vi "PXI4072 Update UI Status.vi"(8 "error in (no error)":errorcluster, 10 "Instr Status":string, 11 "PXI4072 All UI Refs":T1) -> (0 "error out":errorcluster)   [LabVIEW 2026]
uses:
  App Types/References/PXI4072 All UI References.ctl
  App Types/References/PXI4072 Boolean UI References.ctl
  App Types/References/PXI4072 String UI References.ctl
  App Types/References/PXI4072 Numeric UI References.ctl
  App Types/References/PXI4072 Other UI Rerences.ctl
  Drivers/PXI4072/Types/PXI4072 Settings.ctl
  <instrlib>/niDMM/nidmm.llb/niDMM Function.ctl
  <instrlib>/niDMM/nidmm.llb/niDMM Resolution in Digits.ctl
  App Types/Globals/PXI4072 UI Global Refs.vi
  Drivers/PXI4072/PXI4072.lvlib
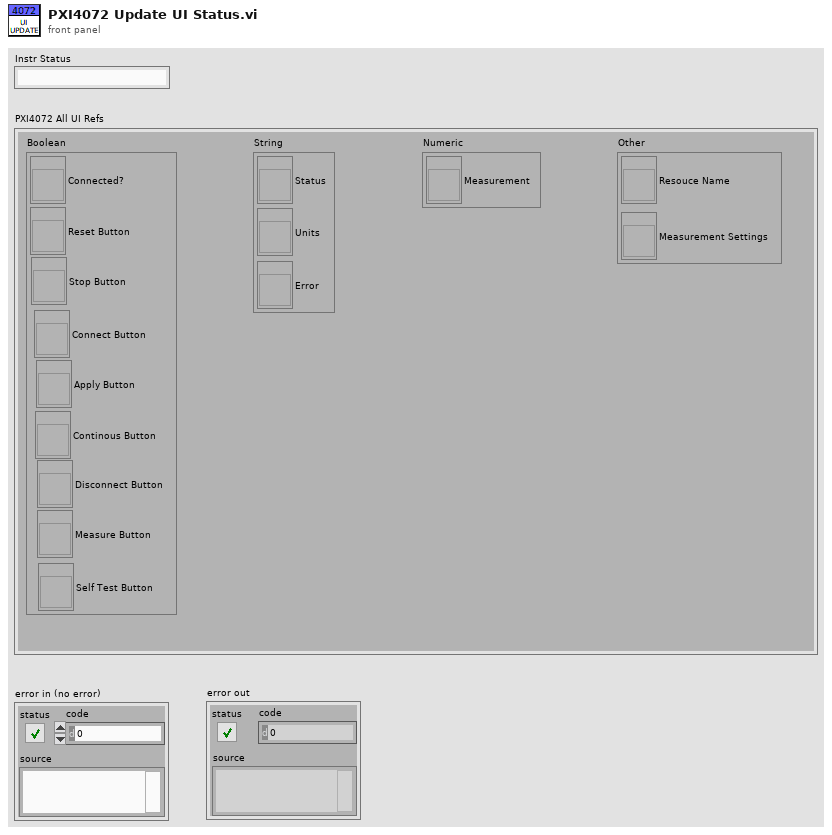
[diagram p1: front panel]
types:
  T1 = typedef "PXI4072 All UI References.ctl" = cluster{"Boolean":T2, "String":T3, "Numeric":T4, "Other":T5}
  T2 = typedef "PXI4072 Boolean UI References.ctl" = cluster{"Connected?":refnum<vi>, "Reset Button":refnum<vi>, "Connect Button":refnum<vi>, "Apply Button":refnum<vi>, "Disconnect Button":refnum<vi>, "Measure Button":refnum<vi>, "Self Test Button":refnum<vi>, "Continous Button":refnum<vi>, "Stop Button":refnum<vi>}
  T3 = typedef "PXI4072 String UI References.ctl" = cluster{"Status":refnum<vi>, "Units":refnum<vi>, "Error":refnum<vi>}
  T4 = typedef "PXI4072 Numeric UI References.ctl" = cluster{"Measurement":refnum<vi>}
  T5 = typedef "PXI4072 Other UI Rerences.ctl" = cluster{"Resouce Name":refnum<vi>, "Measurement Settings":refnum<vi>}
  T6 = enum8{"Enabled", "Disabled", "Disabled and Grayed Out"}
  T7 = typedef "PXI4072.lvlib/PXI4072 Settings.ctl" = cluster{"Function":T8, "Resolution in Digits":T9, "Range":dbl}
  T8 = typedef "niDMM Function.ctl" = enum16{"DC Volts", "AC Volts", "DC Current", "AC Current", "2-wire Resistance", "4-wire Resistance", "Diode", "Frequency", "Period", "AC Volts DC Coupled", "Capacitance", "Inductance", "Temperature"}
  T9 = typedef "niDMM Resolution in Digits.ctl" = dbl
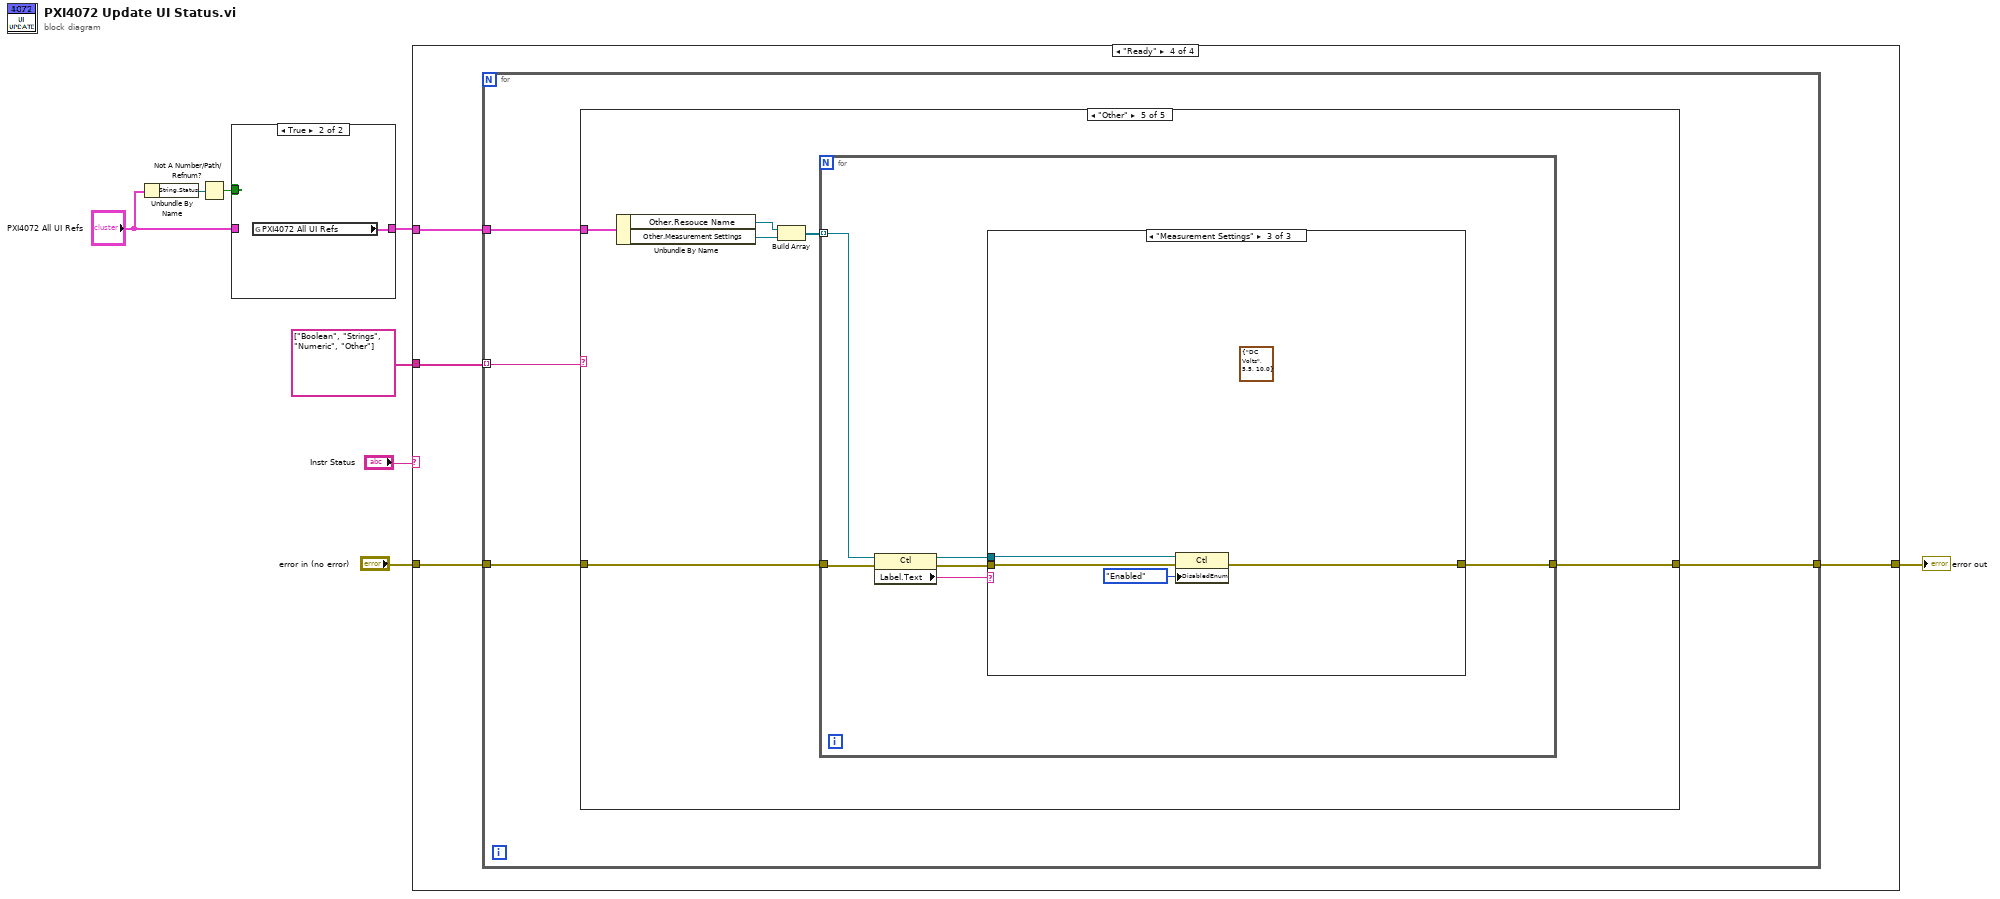
[diagram p0: block diagram]
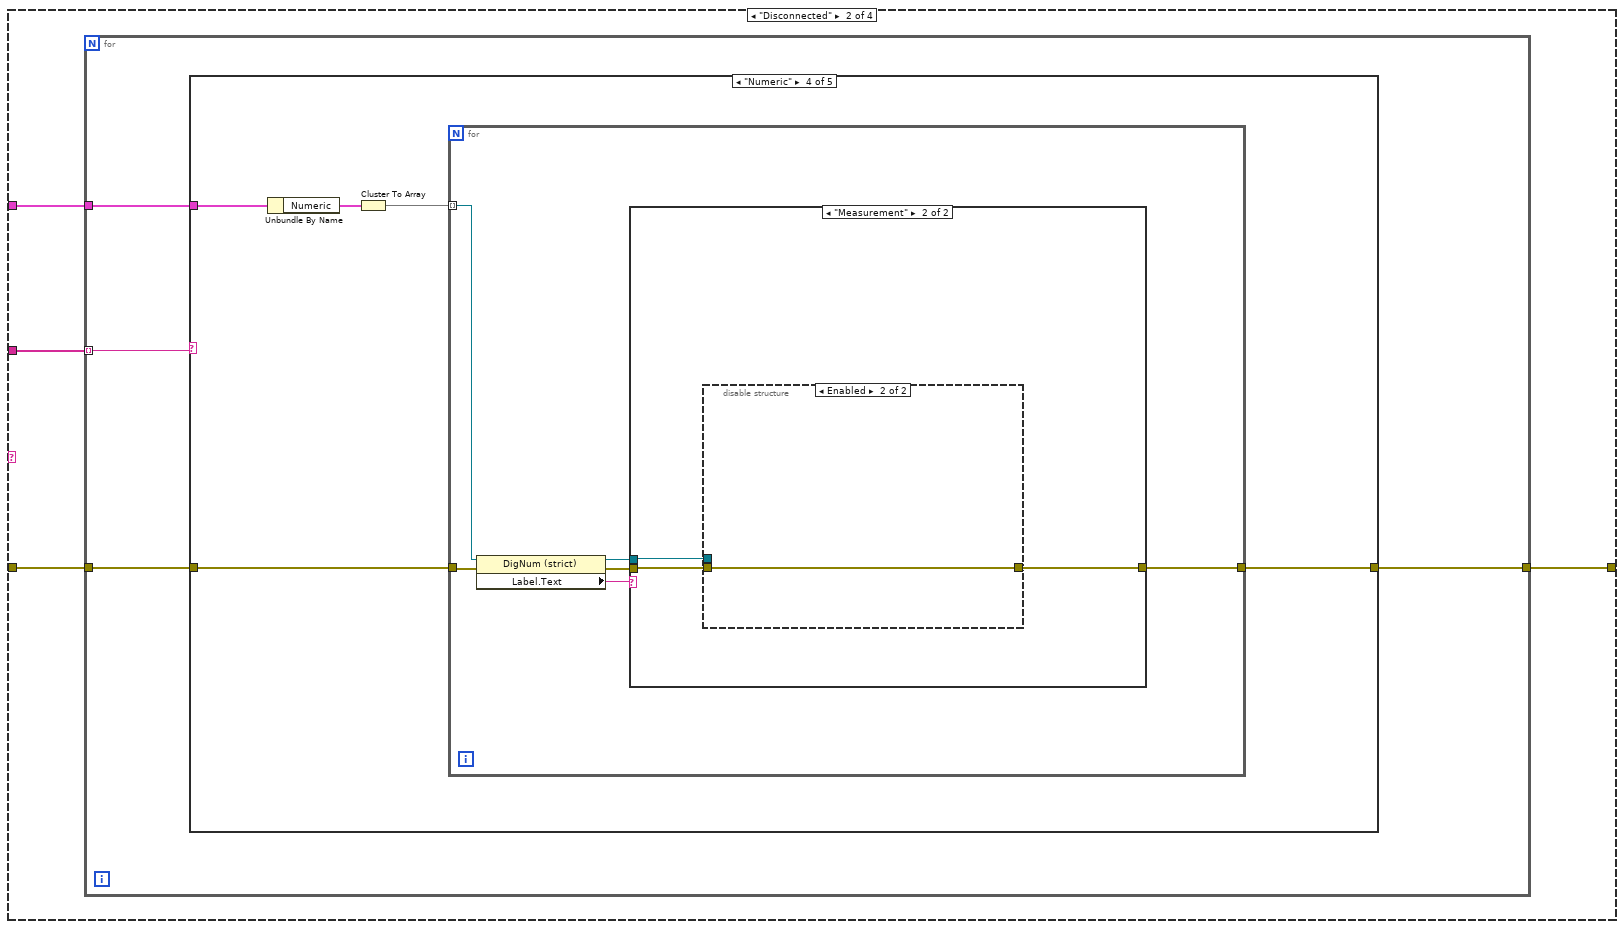
[diagram p4: hidden frame]
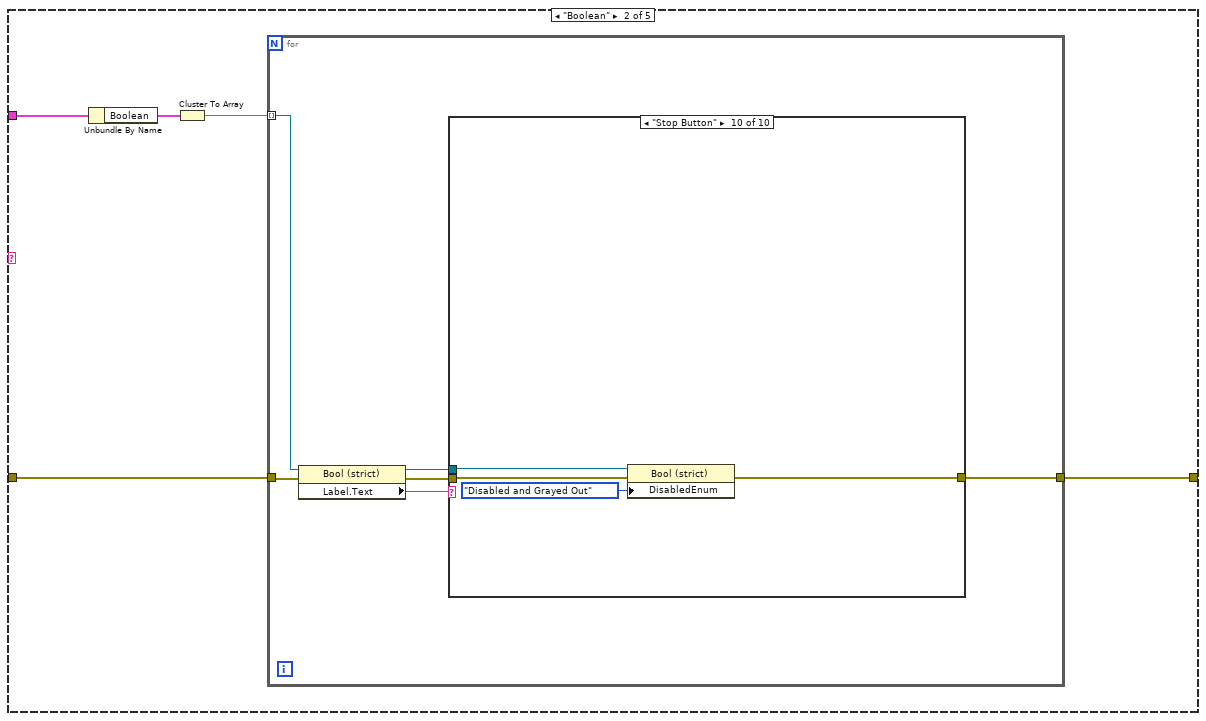
[diagram p6: hidden frame]
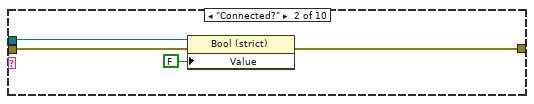
[diagram p8: hidden frame]
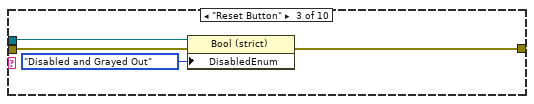
[diagram p9: hidden frame]
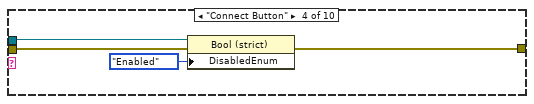
[diagram p10: hidden frame]
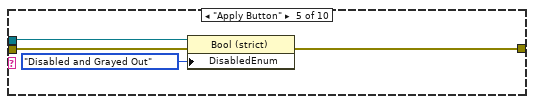
[diagram p11: hidden frame]
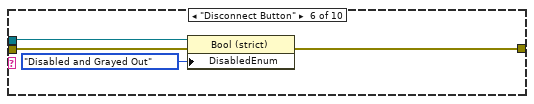
[diagram p12: hidden frame]
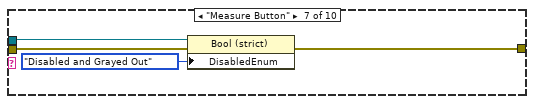
[diagram p13: hidden frame]
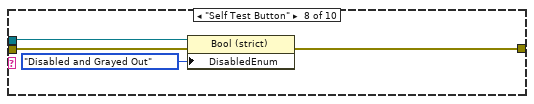
[diagram p14: hidden frame]
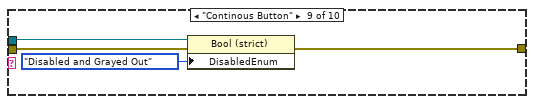
[diagram p15: hidden frame]
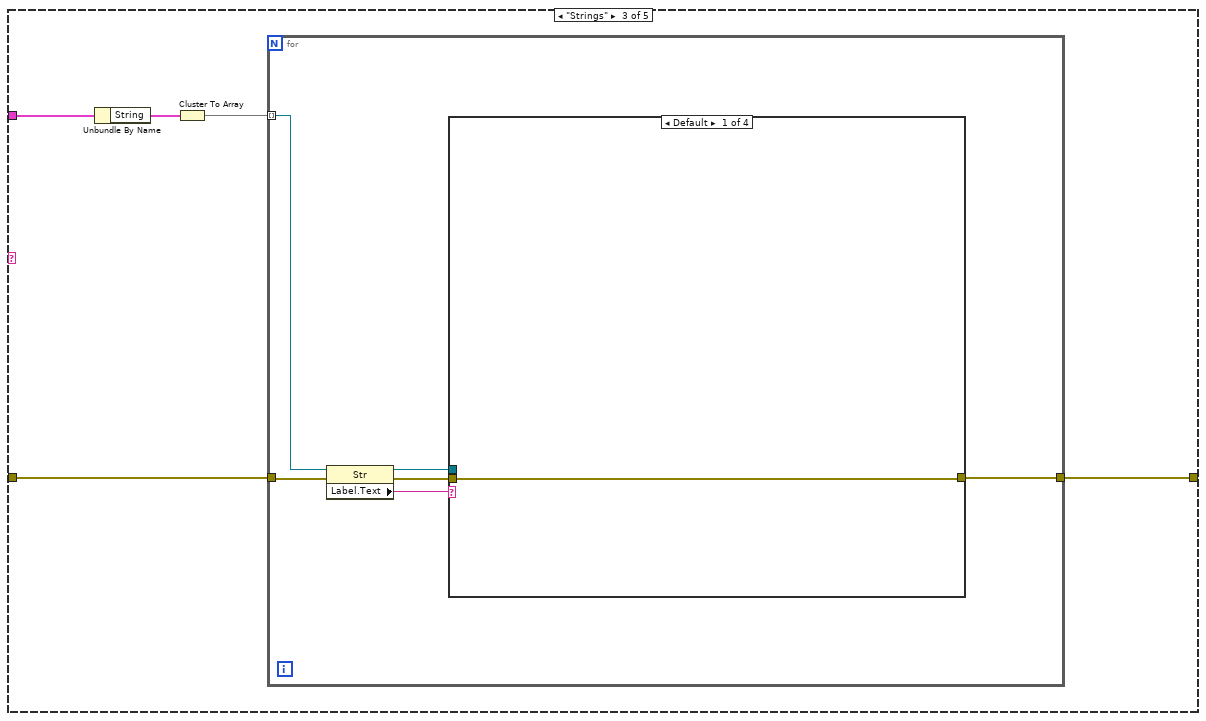
[diagram p16: hidden frame]
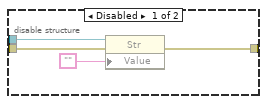
[diagram p18: hidden frame]
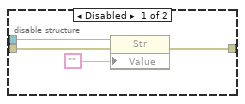
[diagram p20: hidden frame]
diagram:
  n1 = Unbundle By Name("PXI4072 All UI Refs") -> ("String.Status"=w4:refnum<vi>)
  n2 = Not A Number/Path/Refnum?(number/path/refnum=w4) -> (NaN/Path/Refnum?=w1:bool)
  n3 = case shown="True" w1 {
    tunnel: w1 -> [_ _]
    tunnel: "PXI4072 All UI Refs" -> [w9 _]
    tunnel: [w9 w10] -> w2
    frame False {
    }
    frame True, Default {
      n4 = global read "PXI4072 UI Global Refs.vi" "PXI4072 All UI Refs"() -> (w10:T1)
    }
  }
  n5 = case shown="\"Ready\"" "Instr Status" {
    tunnel: string[] ["Boolean", "Strings", "Numeric", "Other"] -> [_ w15 w148 w285]
    tunnel: "error in (no error)" -> [w11 w14 w147 w284]
    tunnel: [w11 w13 w146 w283] -> w6
    tunnel: w2 -> [_ w12 w145 w282]
    frame Default {
    }
    frame "Disconnected" {
      n6 = for {
        tunnel: w15 -> [w19] mode=indexing
        tunnel: w14 -> [w18]
        tunnel: [w17] -> w13
        tunnel: w12 -> [w16]
        n7 = case shown="\"Numeric\"" w19 {
          tunnel: w18 -> [w20 w23 w71 w107 w129]
          tunnel: [w20 w22 w70 w106 w128] -> w17
          tunnel: w16 -> [_ w21 w69 w105 w124]
          frame Default {
          }
          frame "Boolean" {
            n8 = Unbundle By Name(w21) -> ("Boolean"=w25:T2)
            n9 = Cluster To Array(cluster=w25) -> (array=w24:refnum<vi>[])
            n10 = for {
              tunnel: w24 -> [w30] mode=indexing
              tunnel: w23 -> [w31]
              tunnel: [w26] -> w22
              n11 = property class="Bool (strict)"(reference=w30, error in=w31) -> (reference out=w27:refnum<vi>, error out=w29:errorcluster, "Label.Text"=w28:string)
              n12 = case shown="\"Stop Button\"" w28 {
                tunnel: w29 -> [w32 w36 w40 w44 w48 w52 w56 w60 w64 w68]
                tunnel: w27 -> [_ w34 w38 w42 w46 w50 w54 w58 w62 w66]
                tunnel: [w32 w35 w39 w43 w47 w51 w55 w59 w63 w67] -> w26
                frame Default {
                }
                frame "Connected?" {
                  n13 = property class="Bool (strict)"(reference=w34, error in=w36, "Value"=FALSE) -> (error out=w35:errorcluster)  [unwired: 1 out]
                }
                frame "Reset Button" {
                  n14 = property class="Bool (strict)"(reference=w38, error in=w40, "DisabledEnum"=T6."Disabled and Grayed Out" ("Disabled")) -> (error out=w39:errorcluster)  [unwired: 1 out]
                }
                frame "Connect Button" {
                  n15 = property class="Bool (strict)"(reference=w42, error in=w44, "DisabledEnum"=T6."Enabled" ("Disabled")) -> (error out=w43:errorcluster)  [unwired: 1 out]
                }
                frame "Apply Button" {
                  n16 = property class="Bool (strict)"(reference=w46, error in=w48, "DisabledEnum"=T6."Disabled and Grayed Out" ("Disabled")) -> (error out=w47:errorcluster)  [unwired: 1 out]
                }
                frame "Disconnect Button" {
                  n17 = property class="Bool (strict)"(reference=w50, error in=w52, "DisabledEnum"=T6."Disabled and Grayed Out" ("Disabled")) -> (error out=w51:errorcluster)  [unwired: 1 out]
                }
                frame "Measure Button" {
                  n18 = property class="Bool (strict)"(reference=w54, error in=w56, "DisabledEnum"=T6."Disabled and Grayed Out" ("Disabled")) -> (error out=w55:errorcluster)  [unwired: 1 out]
                }
                frame "Self Test Button" {
                  n19 = property class="Bool (strict)"(reference=w58, error in=w60, "DisabledEnum"=T6."Disabled and Grayed Out" ("Disabled")) -> (error out=w59:errorcluster)  [unwired: 1 out]
                }
                frame "Continous Button" {
                  n20 = property class="Bool (strict)"(reference=w62, error in=w64, "DisabledEnum"=T6."Disabled and Grayed Out" ("Disabled")) -> (error out=w63:errorcluster)  [unwired: 1 out]
                }
                frame "Stop Button" {
                  n21 = property class="Bool (strict)"(reference=w66, error in=w68, "DisabledEnum"=T6."Disabled and Grayed Out" ("Disabled")) -> (error out=w67:errorcluster)  [unwired: 1 out]
                }
              }
            }
          }
          frame "Strings" {
            n22 = Unbundle By Name(w69) -> ("String"=w73:T3)
            n23 = Cluster To Array(cluster=w73) -> (array=w72:refnum<vi>[])
            n24 = for {
              tunnel: w72 -> [w78] mode=indexing
              tunnel: w71 -> [w79]
              tunnel: [w74] -> w70
              n25 = property class="Str"(reference=w78, error in=w79) -> (reference out=w75:refnum<vi>, error out=w77:errorcluster, "Label.Text"=w76:string)
              n26 = case shown="Default" w76 {
                tunnel: w77 -> [w80 w83 w91 w99]
                tunnel: w75 -> [_ w81 w89 w97]
                tunnel: [w80 w82 w90 w98] -> w74
                frame Default {
                }
                frame "Status" {
                  n27 = disable-structure shown="Enabled" {
                    disable-tunnel: w83 -> [w87 w88]
                    disable-tunnel: [w86 w88] -> w82
                    disable-tunnel: w81 -> [w85 _]
                    frame Disabled {
                      n28 = property class="Str"(reference=w85, error in=w87, "Value"="") -> (error out=w86:errorcluster)  [unwired: 1 out]
                    }
                    frame Enabled {
                    }
                  }
                }
                frame "Units" {
                  n29 = disable-structure shown="Enabled" {
                    disable-tunnel: w91 -> [w95 w96]
                    disable-tunnel: [w94 w96] -> w90
                    disable-tunnel: w89 -> [w93 _]
                    frame Disabled {
                      n30 = property class="Str"(reference=w93, error in=w95, "Value"="") -> (error out=w94:errorcluster)  [unwired: 1 out]
                    }
                    frame Enabled {
                    }
                  }
                }
                frame "Error" {
                  n31 = disable-structure shown="Enabled" {
                    disable-tunnel: w99 -> [w103 w104]
                    disable-tunnel: [w102 w104] -> w98
                    disable-tunnel: w97 -> [w101 _]
                    frame Disabled {
                      n32 = property class="Str"(reference=w101, error in=w103, "Value"="") -> (error out=w102:errorcluster)  [unwired: 1 out]
                    }
                    frame Enabled {
                    }
                  }
                }
              }
            }
          }
          frame "Numeric" {
            n33 = Unbundle By Name(w105) -> ("Numeric"=w109:T4)
            n34 = Cluster To Array(cluster=w109) -> (array=w108:refnum<vi>[])
            n35 = for {
              tunnel: w108 -> [w114] mode=indexing
              tunnel: w107 -> [w115]
              tunnel: [w110] -> w106
              n36 = property class="DigNum (strict)"(reference=w114, error in=w115) -> (reference out=w111:refnum<vi>, error out=w113:errorcluster, "Label.Text"=w112:string)
              n37 = case shown="\"Measurement\"" w112 {
                tunnel: w113 -> [w116 w119]
                tunnel: w111 -> [_ w117]
                tunnel: [w116 w118] -> w110
                frame Default {
                }
                frame "Measurement" {
                  n38 = disable-structure shown="Enabled" {
                    disable-tunnel: w119 -> [w122 w123]
                    disable-tunnel: [w121 w123] -> w118
                    disable-tunnel: w117 -> [w120 _]
                    frame Disabled {
                      n39 = property class="DigNum (strict)" props=["DisabledEnum"](reference=w120, error in=w122) -> (error out=w121:errorcluster)  [unwired: 1 in, 1 out]
                    }
                    frame Enabled {
                    }
                  }
                }
              }
            }
          }
          frame "Other" {
            n40 = Unbundle By Name(w124) -> ("Other.Resouce Name"=w127:refnum<vi>, "Other.Measurement Settings"=w126:refnum<vi>)
            n41 = Build Array(w127, w126) -> (w125:refnum<vi>[])
            n42 = for {
              tunnel: w129 -> [w135]
              tunnel: [w131] -> w128
              tunnel: w125 -> [w130] mode=indexing
              n43 = property class="Ctl"(reference=w130, error in=w135) -> (reference out=w132:refnum<vi>, error out=w134:errorcluster, "Label.Text"=w133:string)
              n44 = case shown="\"Measurement Settings\"" w133 {
                tunnel: w134 -> [w136 w140 w144]
                tunnel: w132 -> [_ w138 w142]
                tunnel: [w136 w139 w143] -> w131
                frame Default {
                }
                frame "Resource Name" {
                  n45 = property class="Ctl"(reference=w138, error in=w140, "DisabledEnum"=T6."Enabled" ("Disabled")) -> (error out=w139:errorcluster)  [unwired: 1 out]
                }
                frame "Measurement Settings" {
                  (unwired) T7 {"Function"=enum."DC Volts", "Resolution in Digits"=5.5, "Range"=10.0} ("Measurement Settings")
                  n46 = property class="Ctl"(reference=w142, error in=w144, "DisabledEnum"=T6."Disabled and Grayed Out" ("Disabled")) -> (error out=w143:errorcluster)  [unwired: 1 out]
                }
              }
            }
          }
        }
      }
    }
    frame "Connected" {
      n47 = for {
        tunnel: w148 -> [w152] mode=indexing
        tunnel: w147 -> [w151]
        tunnel: [w150] -> w146
        tunnel: w145 -> [w149]
        n48 = case shown="\"Other\"" w152 {
          tunnel: w151 -> [w153 w156 w208 w244 w266]
          tunnel: [w153 w155 w207 w243 w265] -> w150
          tunnel: w149 -> [_ w154 w206 w242 w261]
          frame Default {
          }
          frame "Boolean" {
            n49 = Unbundle By Name(w154) -> ("Boolean"=w158:T2)
            n50 = Cluster To Array(cluster=w158) -> (array=w157:refnum<vi>[])
            n51 = for {
              tunnel: w157 -> [w163] mode=indexing
              tunnel: w156 -> [w164]
              tunnel: [w159] -> w155
              n52 = property class="Bool (strict)"(reference=w163, error in=w164) -> (reference out=w160:refnum<vi>, error out=w162:errorcluster, "Label.Text"=w161:string)
              n53 = case shown="\"Measure Button\"" w161 {
                tunnel: w162 -> [w165 w168 w177 w181 w185 w189 w193 w197 w201 w205]
                tunnel: w160 -> [_ w166 w175 w179 w183 w187 w191 w195 w199 w203]
                tunnel: [w165 w167 w176 w180 w184 w188 w192 w196 w200 w204] -> w159
                frame Default {
                }
                frame "Connected?" {
                  n54 = disable-structure shown="Enabled" {
                    disable-tunnel: w168 -> [w172 w173]
                    disable-tunnel: [w171 w173] -> w167
                    disable-tunnel: w166 -> [w170 _]
                    frame Disabled {
                      n55 = property class="Bool (strict)"(reference=w170, error in=w172, "Value"=FALSE) -> (error out=w171:errorcluster)  [unwired: 1 out]
                    }
                    frame Enabled {
                    }
                  }
                }
                frame "Reset Button" {
                  n56 = property class="Bool (strict)"(reference=w175, error in=w177, "DisabledEnum"=T6."Enabled" ("Disabled")) -> (error out=w176:errorcluster)  [unwired: 1 out]
                }
                frame "Connect Button" {
                  n57 = property class="Bool (strict)"(reference=w179, error in=w181, "DisabledEnum"=T6."Disabled and Grayed Out" ("Disabled")) -> (error out=w180:errorcluster)  [unwired: 1 out]
                }
                frame "Apply Button" {
                  n58 = property class="Bool (strict)"(reference=w183, error in=w185, "DisabledEnum"=T6."Enabled" ("Disabled")) -> (error out=w184:errorcluster)  [unwired: 1 out]
                }
                frame "Disconnect Button" {
                  n59 = property class="Bool (strict)"(reference=w187, error in=w189, "DisabledEnum"=T6."Enabled" ("Disabled")) -> (error out=w188:errorcluster)  [unwired: 1 out]
                }
                frame "Measure Button" {
                  n60 = property class="Bool (strict)"(reference=w191, error in=w193, "DisabledEnum"=T6."Disabled and Grayed Out" ("Disabled")) -> (error out=w192:errorcluster)  [unwired: 1 out]
                }
                frame "Self Test Button" {
                  n61 = property class="Bool (strict)"(reference=w195, error in=w197, "DisabledEnum"=T6."Enabled" ("Disabled")) -> (error out=w196:errorcluster)  [unwired: 1 out]
                }
                frame "Continous Button" {
                  n62 = property class="Bool (strict)"(reference=w199, error in=w201, "DisabledEnum"=T6."Disabled and Grayed Out" ("Disabled")) -> (error out=w200:errorcluster)  [unwired: 1 out]
                }
                frame "Stop Button" {
                  n63 = property class="Bool (strict)"(reference=w203, error in=w205, "DisabledEnum"=T6."Disabled and Grayed Out" ("Disabled")) -> (error out=w204:errorcluster)  [unwired: 1 out]
                }
              }
            }
          }
          frame "Strings" {
            n64 = Unbundle By Name(w206) -> ("String"=w210:T3)
            n65 = Cluster To Array(cluster=w210) -> (array=w209:refnum<vi>[])
            n66 = for {
              tunnel: w209 -> [w215] mode=indexing
              tunnel: w208 -> [w216]
              tunnel: [w211] -> w207
              n67 = property class="Str"(reference=w215, error in=w216) -> (reference out=w212:refnum<vi>, error out=w214:errorcluster, "Label.Text"=w213:string)
              n68 = case shown="Default" w213 {
                tunnel: w214 -> [w217 w220 w228 w236]
                tunnel: w212 -> [_ w218 w226 w234]
                tunnel: [w217 w219 w227 w235] -> w211
                frame Default {
                }
                frame "Status" {
                  n69 = disable-structure shown="Enabled" {
                    disable-tunnel: w220 -> [w224 w225]
                    disable-tunnel: [w223 w225] -> w219
                    disable-tunnel: w218 -> [w222 _]
                    frame Disabled {
                      n70 = property class="Str"(reference=w222, error in=w224, "Value"="") -> (error out=w223:errorcluster)  [unwired: 1 out]
                    }
                    frame Enabled {
                    }
                  }
                }
                frame "Units" {
                  n71 = disable-structure shown="Enabled" {
                    disable-tunnel: w228 -> [w232 w233]
                    disable-tunnel: [w231 w233] -> w227
                    disable-tunnel: w226 -> [w230 _]
                    frame Disabled {
                      n72 = property class="Str"(reference=w230, error in=w232, "Value"="") -> (error out=w231:errorcluster)  [unwired: 1 out]
                    }
                    frame Enabled {
                    }
                  }
                }
                frame "Error" {
                  n73 = disable-structure shown="Enabled" {
                    disable-tunnel: w236 -> [w240 w241]
                    disable-tunnel: [w239 w241] -> w235
                    disable-tunnel: w234 -> [w238 _]
                    frame Disabled {
                      n74 = property class="Str"(reference=w238, error in=w240, "Value"="") -> (error out=w239:errorcluster)  [unwired: 1 out]
                    }
                    frame Enabled {
                    }
                  }
                }
              }
            }
          }
          frame "Numeric" {
            n75 = Unbundle By Name(w242) -> ("Numeric"=w246:T4)
            n76 = Cluster To Array(cluster=w246) -> (array=w245:refnum<vi>[])
            n77 = for {
              tunnel: w245 -> [w251] mode=indexing
              tunnel: w244 -> [w252]
              tunnel: [w247] -> w243
              n78 = property class="DigNum (strict)"(reference=w251, error in=w252) -> (reference out=w248:refnum<vi>, error out=w250:errorcluster, "Label.Text"=w249:string)
              n79 = case shown="\"Measurement\"" w249 {
                tunnel: w250 -> [w253 w256]
                tunnel: w248 -> [_ w254]
                tunnel: [w253 w255] -> w247
                frame Default {
                }
                frame "Measurement" {
                  n80 = disable-structure shown="Enabled" {
                    disable-tunnel: w256 -> [w259 w260]
                    disable-tunnel: [w258 w260] -> w255
                    disable-tunnel: w254 -> [w257 _]
                    frame Disabled {
                      n81 = property class="DigNum (strict)" props=["DisabledEnum"](reference=w257, error in=w259) -> (error out=w258:errorcluster)  [unwired: 1 in, 1 out]
                    }
                    frame Enabled {
                    }
                  }
                }
              }
            }
          }
          frame "Other" {
            n82 = Unbundle By Name(w261) -> ("Other.Resouce Name"=w264:refnum<vi>, "Other.Measurement Settings"=w263:refnum<vi>)
            n83 = Build Array(w264, w263) -> (w262:refnum<vi>[])
            n84 = for {
              tunnel: w266 -> [w272]
              tunnel: [w268] -> w265
              tunnel: w262 -> [w267] mode=indexing
              n85 = property class="Ctl"(reference=w267, error in=w272) -> (reference out=w269:refnum<vi>, error out=w271:errorcluster, "Label.Text"=w270:string)
              n86 = case shown="\"Measurement Settings\"" w270 {
                tunnel: w271 -> [w273 w277 w281]
                tunnel: w269 -> [_ w275 w279]
                tunnel: [w273 w276 w280] -> w268
                frame Default {
                }
                frame "Resource Name" {
                  n87 = property class="Ctl"(reference=w275, error in=w277, "DisabledEnum"=T6."Disabled and Grayed Out" ("Disabled")) -> (error out=w276:errorcluster)  [unwired: 1 out]
                }
                frame "Measurement Settings" {
                  (unwired) T7 {"Function"=enum."DC Volts", "Resolution in Digits"=5.5, "Range"=10.0} ("Measurement Settings")
                  n88 = property class="Ctl"(reference=w279, error in=w281, "DisabledEnum"=T6."Enabled" ("Disabled")) -> (error out=w280:errorcluster)  [unwired: 1 out]
                }
              }
            }
          }
        }
      }
    }
    frame "Ready" {
      n89 = for {
        tunnel: w285 -> [w289] mode=indexing
        tunnel: w284 -> [w288]
        tunnel: [w287] -> w283
        tunnel: w282 -> [w286]
        n90 = case shown="\"Other\"" w289 {
          tunnel: w288 -> [w290 w293 w345 w381 w403]
          tunnel: [w290 w292 w344 w380 w402] -> w287
          tunnel: w286 -> [_ w291 w343 w379 w398]
          frame Default {
          }
          frame "Boolean" {
            n91 = Unbundle By Name(w291) -> ("Boolean"=w295:T2)
            n92 = Cluster To Array(cluster=w295) -> (array=w294:refnum<vi>[])
            n93 = for {
              tunnel: w294 -> [w300] mode=indexing
              tunnel: w293 -> [w301]
              tunnel: [w296] -> w292
              n94 = property class="Bool (strict)"(reference=w300, error in=w301) -> (reference out=w297:refnum<vi>, error out=w299:errorcluster, "Label.Text"=w298:string)
              n95 = case shown="\"Connect Button\"" w298 {
                tunnel: w299 -> [w302 w305 w314 w318 w322 w326 w330 w334 w338 w342]
                tunnel: w297 -> [_ w303 w312 w316 w320 w324 w328 w332 w336 w340]
                tunnel: [w302 w304 w313 w317 w321 w325 w329 w333 w337 w341] -> w296
                frame Default {
                }
                frame "Connected?" {
                  n96 = disable-structure shown="Enabled" {
                    disable-tunnel: w305 -> [w309 w310]
                    disable-tunnel: [w308 w310] -> w304
                    disable-tunnel: w303 -> [w307 _]
                    frame Disabled {
                      n97 = property class="Bool (strict)"(reference=w307, error in=w309, "Value"=FALSE) -> (error out=w308:errorcluster)  [unwired: 1 out]
                    }
                    frame Enabled {
                    }
                  }
                }
                frame "Reset Button" {
                  n98 = property class="Bool (strict)"(reference=w312, error in=w314, "DisabledEnum"=T6."Enabled" ("Disabled")) -> (error out=w313:errorcluster)  [unwired: 1 out]
                }
                frame "Connect Button" {
                  n99 = property class="Bool (strict)"(reference=w316, error in=w318, "DisabledEnum"=T6."Disabled and Grayed Out" ("Disabled")) -> (error out=w317:errorcluster)  [unwired: 1 out]
                }
                frame "Apply Button" {
                  n100 = property class="Bool (strict)"(reference=w320, error in=w322, "DisabledEnum"=T6."Enabled" ("Disabled")) -> (error out=w321:errorcluster)  [unwired: 1 out]
                }
                frame "Disconnect Button" {
                  n101 = property class="Bool (strict)"(reference=w324, error in=w326, "DisabledEnum"=T6."Enabled" ("Disabled")) -> (error out=w325:errorcluster)  [unwired: 1 out]
                }
                frame "Measure Button" {
                  n102 = property class="Bool (strict)"(reference=w328, error in=w330, "DisabledEnum"=T6."Enabled" ("Disabled")) -> (error out=w329:errorcluster)  [unwired: 1 out]
                }
                frame "Self Test Button" {
                  n103 = property class="Bool (strict)"(reference=w332, error in=w334, "DisabledEnum"=T6."Enabled" ("Disabled")) -> (error out=w333:errorcluster)  [unwired: 1 out]
                }
                frame "Continous Button" {
                  n104 = property class="Bool (strict)"(reference=w336, error in=w338, "DisabledEnum"=T6."Enabled" ("Disabled")) -> (error out=w337:errorcluster)  [unwired: 1 out]
                }
                frame "Stop Button" {
                  n105 = property class="Bool (strict)"(reference=w340, error in=w342, "DisabledEnum"=T6."Enabled" ("Disabled")) -> (error out=w341:errorcluster)  [unwired: 1 out]
                }
              }
            }
          }
          frame "Strings" {
            n106 = Unbundle By Name(w343) -> ("String"=w347:T3)
            n107 = Cluster To Array(cluster=w347) -> (array=w346:refnum<vi>[])
            n108 = for {
              tunnel: w346 -> [w352] mode=indexing
              tunnel: w345 -> [w353]
              tunnel: [w348] -> w344
              n109 = property class="Str"(reference=w352, error in=w353) -> (reference out=w349:refnum<vi>, error out=w351:errorcluster, "Label.Text"=w350:string)
              n110 = case shown="Default" w350 {
                tunnel: w351 -> [w354 w357 w365 w373]
                tunnel: w349 -> [_ w355 w363 w371]
                tunnel: [w354 w356 w364 w372] -> w348
                frame Default {
                }
                frame "Status" {
                  n111 = disable-structure shown="Enabled" {
                    disable-tunnel: w357 -> [w361 w362]
                    disable-tunnel: [w360 w362] -> w356
                    disable-tunnel: w355 -> [w359 _]
                    frame Disabled {
                      n112 = property class="Str"(reference=w359, error in=w361, "Value"="") -> (error out=w360:errorcluster)  [unwired: 1 out]
                    }
                    frame Enabled {
                    }
                  }
                }
                frame "Units" {
                  n113 = disable-structure shown="Enabled" {
                    disable-tunnel: w365 -> [w369 w370]
                    disable-tunnel: [w368 w370] -> w364
                    disable-tunnel: w363 -> [w367 _]
                    frame Disabled {
                      n114 = property class="Str"(reference=w367, error in=w369, "Value"="") -> (error out=w368:errorcluster)  [unwired: 1 out]
                    }
                    frame Enabled {
                    }
                  }
                }
                frame "Error" {
                  n115 = disable-structure shown="Enabled" {
                    disable-tunnel: w373 -> [w377 w378]
                    disable-tunnel: [w376 w378] -> w372
                    disable-tunnel: w371 -> [w375 _]
                    frame Disabled {
                      n116 = property class="Str"(reference=w375, error in=w377, "Value"="") -> (error out=w376:errorcluster)  [unwired: 1 out]
                    }
                    frame Enabled {
                    }
                  }
                }
              }
            }
          }
          frame "Numeric" {
            n117 = Unbundle By Name(w379) -> ("Numeric"=w383:T4)
            n118 = Cluster To Array(cluster=w383) -> (array=w382:refnum<vi>[])
            n119 = for {
              tunnel: w382 -> [w388] mode=indexing
              tunnel: w381 -> [w389]
              tunnel: [w384] -> w380
              n120 = property class="DigNum (strict)"(reference=w388, error in=w389) -> (reference out=w385:refnum<vi>, error out=w387:errorcluster, "Label.Text"=w386:string)
              n121 = case shown="\"Measurement\"" w386 {
                tunnel: w387 -> [w390 w393]
                tunnel: w385 -> [_ w391]
                tunnel: [w390 w392] -> w384
                frame Default {
                }
                frame "Measurement" {
                  n122 = disable-structure shown="Enabled" {
                    disable-tunnel: w393 -> [w396 w397]
                    disable-tunnel: [w395 w397] -> w392
                    disable-tunnel: w391 -> [w394 _]
                    frame Disabled {
                      n123 = property class="DigNum (strict)" props=["DisabledEnum"](reference=w394, error in=w396) -> (error out=w395:errorcluster)  [unwired: 1 in, 1 out]
                    }
                    frame Enabled {
                    }
                  }
                }
              }
            }
          }
          frame "Other" {
            n124 = Unbundle By Name(w398) -> ("Other.Resouce Name"=w401:refnum<vi>, "Other.Measurement Settings"=w400:refnum<vi>)
            n125 = Build Array(w401, w400) -> (w399:refnum<vi>[])
            n126 = for {
              tunnel: w403 -> [w409]
              tunnel: [w405] -> w402
              tunnel: w399 -> [w404] mode=indexing
              n127 = property class="Ctl"(reference=w404, error in=w409) -> (reference out=w406:refnum<vi>, error out=w408:errorcluster, "Label.Text"=w407:string)
              n128 = case shown="\"Measurement Settings\"" w407 {
                tunnel: w408 -> [w410 w414 w418]
                tunnel: w406 -> [_ w412 w416]
                tunnel: [w410 w413 w417] -> w405
                frame Default {
                }
                frame "Resource Name" {
                  n129 = property class="Ctl"(reference=w412, error in=w414, "DisabledEnum"=T6."Disabled and Grayed Out" ("Disabled")) -> (error out=w413:errorcluster)  [unwired: 1 out]
                }
                frame "Measurement Settings" {
                  (unwired) T7 {"Function"=enum."DC Volts", "Resolution in Digits"=5.5, "Range"=10.0} ("Measurement Settings")
                  n130 = property class="Ctl"(reference=w416, error in=w418, "DisabledEnum"=T6."Enabled" ("Disabled")) -> (error out=w417:errorcluster)  [unwired: 1 out]
                }
              }
            }
          }
        }
      }
    }
  }
  "error out" <- w6
